vi "SVPO Scale Voltage to EU (N Ch - N Info SGL Array).vi"(10 "channel info":T1[](array[typedef]) {"pregain" format="%.2f"; "weighting filter" items=["Linear", "A-weighting", "B-weighting", "C-weighting", "ITU-R 468-4", "Dolby", "CCITT", "C-message", "Wb", "Wc", "Wd", "We", "Wf", "Wh", "Wj", "Wk", "Wm", "AES17 20 kHz lowpass", "AES17 40 kHz lowpass", "AES17 20 kHz highpass", "AES17 40 kHz highpass"]; "dB reference" format="%^.1e"; "engineering units" items=["custom..."=0, "V"=1, "A"=21, "C"=30, "pC"=31, "s"=32, "-"=29, "Pa"=2, "N"=20, "g"=3, "m/s^2"=4, "m/s"=5, "m"=6, "mm/s"=12, "mm"=13, "micron/s"=14, "micron"=15, "in/s^2"=7, "in/s"=8, "in"=9, "mil/s"=10, "mil"=11, "rad/s^2"=16, "rad/s"=17, "rad"=18, "deg/s^2"=26, "deg/s"=27, "deg"=28, "RPM"=22, "cycle/s^2"=23, "Hz"=24, "cycle"=25, "strain"=19]; "sensor sensitivity" format="%#_5f"}, 11 "signals [V]":sgl[][](array[numeric])) -> (2 "unit labels":string[](array[string]), 3 "scaled signals [EU]":sgl[][](array[numeric]))   [LabVIEW 2017, in "SoundVib_Calibration.lvlib"]
doc: "Scales the single-precision <B>signal [V]</B> from volts to the engineering units (EU) you select. Scale signals to appropriate EU before applying limits, saving to disk, and performing measurement analyses. Use this VI on embedded targets that have limited computational resources. Wire data to the <B>signal [V]</B> input to determine the polymorphic instance to use or manually select the instance."
uses:
  <vilib>/addons/Sound and Vibration/svt_Calibration/SoundVib_Calibration.lvlib
  <vilib>/addons/_NISVFA/_Shared subVIs/Controls/svc_Channel Info.ctl
  <vilib>/addons/_NISVFA/_Shared subVIs/Controls/svc_Engineering Units Text Ring.ctl
  <vilib>/addons/_NISVFA/_Shared subVIs/Controls/svc_Weighting Filter Text Ring.ctl
  <vilib>/addons/_NISVFA/_Shared subVIs/Common/svc_Compute Scale Factor to Convert V to EU.vi
  <vilib>/addons/_NISVFA/_Shared subVIs/Common/svc_Engineering Units to Unit Label.vi
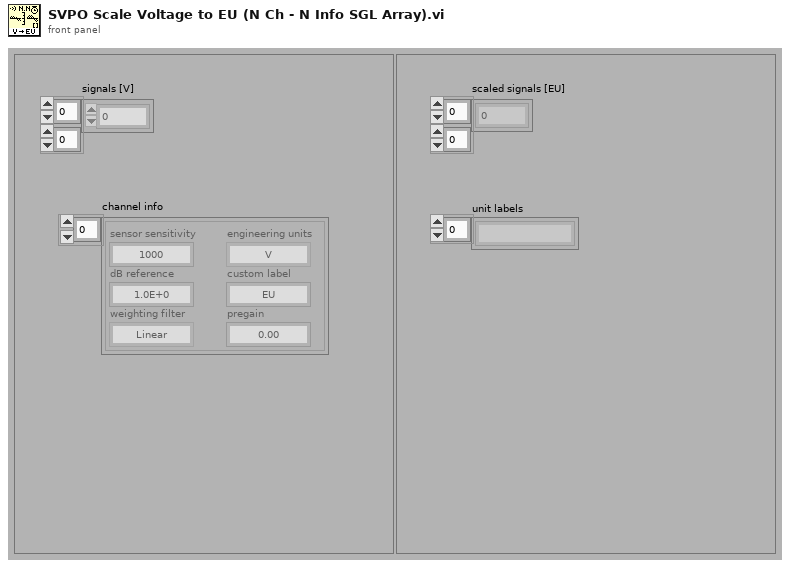
[diagram p1: front panel]
types:
  T1 = typedef "svc_Channel Info.ctl" = cluster{"sensor sensitivity":dbl, "engineering units":T2, "dB reference":dbl, "custom label":string, "weighting filter":T3, "pregain":dbl}
  T2 = typedef "svc_Engineering Units Text Ring.ctl" = u16
  T3 = typedef "svc_Weighting Filter Text Ring.ctl" = u16
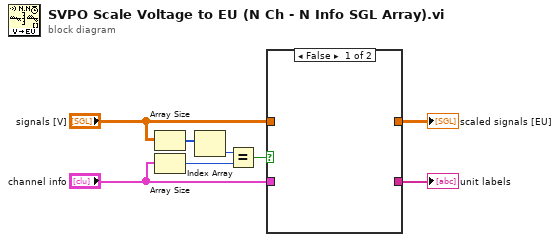
[diagram p0: block diagram]
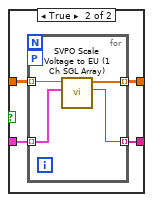
[diagram p2: hidden frame]
diagram:
  n1 = Array Size(array="signals [V]") -> (size(s)=w4:i32[])
  n2 = Array Size(array="channel info") -> (size(s)=w7:i32)
  n3 = Index Array(array=w4) -> (element=w3:i32)  [unwired: 1 in]
  n4 = Equal?(x=w3, y=w7) -> (x = y?=w2:bool)
  n5 = case shown="False" w2 {
    tunnel: [_ w12] -> w8
    tunnel: [_ w11] -> w1
    tunnel: "signals [V]" -> [_ w10]
    tunnel: "channel info" -> [_ w9]
    frame False {
    }
    frame True {
      n6 = for {
        tunnel: w10 -> [w16] mode=indexing
        tunnel: w9 -> [w15] mode=indexing
        tunnel: [w14] -> w12 mode=indexing
        tunnel: [w13] -> w11 mode=indexing
        workers-P: _ -> [_]
        n7 = call <vilib>:"SVPO Scale Voltage to EU (1 Ch SGL Array).vi"("channel info"=w15, "signal [V]"=w16) -> ("unit label"=w13:string, "scaled signal [EU]"=w14:sgl[])  [unwired: 8 in]
      }
    }
  }
  "scaled signals [EU]" <- w8
  "unit labels" <- w1
